vi "Test_Determination_of_Min_Max_Average_Value.vi"() -> ()   [LabVIEW 2022 SP3]
uses:
  SI_modules/SI600/SI600.lvclass
panel:
  out "RCP Spped Loop":cluster{"Time":timestamp[], dbl[]}[](graph)
  out "Inputs":cluster{"Time":timestamp[], dbl[]}[](graph)
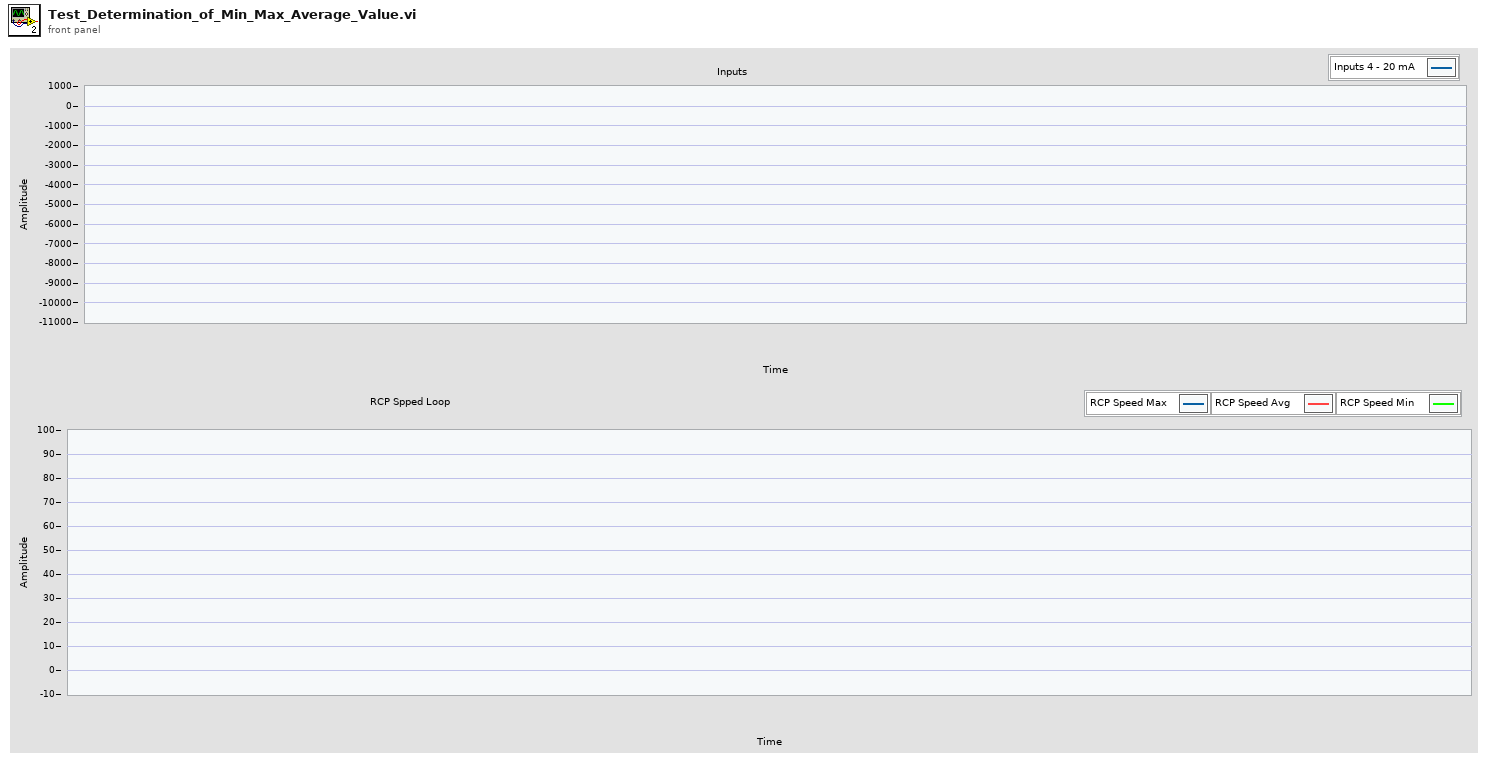
[diagram p1: front panel]
types:
  T1 = cluster{"[0]":cluster{"Time":timestamp[], "KKS":string, "Meas":dbl[]}, "[1]":cluster{"Time":timestamp[], "KKS":string, "Meas":dbl[]}, "[2]":cluster{"Time":timestamp[], "KKS":string, "Meas":dbl[]}, "[3]":cluster{"Time":timestamp[], "KKS":string, "Meas":dbl[]}, "[4]":cluster{"Time":timestamp[], "KKS":string, "Meas":dbl[]}, "[5]":cluster{"Time":timestamp[], "KKS":string, "Meas":dbl[]}, "[6]":cluster{"Time":timestamp[], "KKS":string, "Meas":dbl[]}, "[7]":cluster{"Time":timestamp[], "KKS":string, "Meas":dbl[]}, "[8]":cluster{"Time":timestamp[], "KKS":string, "Meas":dbl[]}}
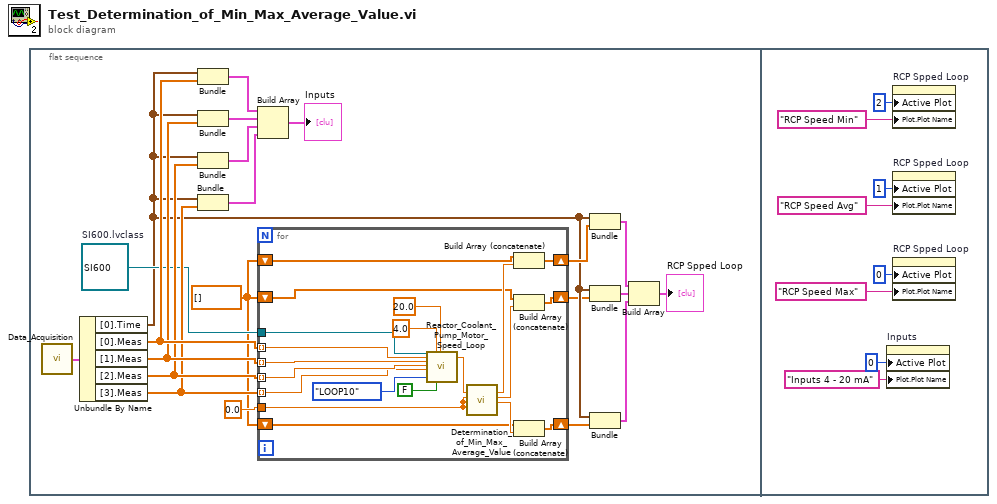
[diagram p0: block diagram]
diagram:
  n1 = flat-sequence {
    frame #0 {
      w11 = refnum<class "SI600.lvclass"> refnum  # SI600.lvclass
      w9 = dbl[] []
      n2 = call "Data_Acquisition.vi"() -> ("Meas"=w21:T1)  [unwired: 15 in]
      n3 = Unbundle By Name(w21) -> ("[0].Time"=w7:timestamp[], "[0].Meas"=w20:dbl[], "[1].Meas"=w19:dbl[], "[2].Meas"=w18:dbl[], "[3].Meas"=w17:dbl[])
      n4 = Bundle("Time"=w7, "Meas"=w20) -> (w16:cluster{"Time":timestamp[], "Meas":dbl[]})  [unwired: 1 in]
      n5 = Bundle("Time"=w7, "Meas"=w19) -> (w15:cluster{"Time":timestamp[], "Meas":dbl[]})  [unwired: 1 in]
      n6 = Bundle("Time"=w7, "Meas"=w18) -> (w14:cluster{"Time":timestamp[], "Meas":dbl[]})  [unwired: 1 in]
      n7 = Bundle("Time"=w7, "Meas"=w17) -> (w13:cluster{"Time":timestamp[], "Meas":dbl[]})  [unwired: 1 in]
      n8 = Build Array(w16, w15, w14, w13) -> (→"Inputs":cluster{"Time":timestamp[], "Meas":dbl[]}[])
      n9 = for {
        tunnel: w11 -> [w41]
        tunnel: w20 -> [w40] mode=indexing
        tunnel: w19 -> [w39] mode=indexing
        tunnel: w18 -> [w38] mode=indexing
        tunnel: w17 -> [w37] mode=indexing
        tunnel: 0.0 ("RCP speed Loop 20") -> [w31]
        shift-right: [w27] -> w8
        shift-left: w9 -> [w24]
        shift-right: [w26] -> w6
        shift-left: w9 -> [w23]
        shift-right: [w25] -> w5
        shift-left: w9 -> [w22]
        n10 = call "Reactor_Coolant_Pump_Motor_Speed_Loop.vi"("SI600.lvclass in"=w41, "3 JEB CS951 XQ01"=w40, "3 JEB CS952 XQ01"=w39, "3 JEB CS953 XQ01"=w38, "3 JEB CS954 XQ01"=w37, "Loop"=enum16{"LOOP10", "LOOP20", "LOOP30", "LOOP40"}."LOOP10", "In1"=4.0, "Limitation"=FALSE, "In2"=20.0) -> ("RCP speed Loop Output"=w32:dbl)  [unwired: 12 in, 6 out]
        n11 = call "Determination_of_Min_Max_Average_Value.vi"("RCP speed Loop 10"=w32, "RCP speed Loop 20"=w31, "RCP speed Loop 30"=w31, "RCP speed Loop 40"=w31) -> ("RCP Speed Max"=w30:dbl, "RCP Speed AVG"=w29:dbl, "RCP Speed Min"=w28:dbl)  [unwired: 11 in, 2 out]
        n12 = Build Array (concatenate)(w24, w30) -> (w27:dbl[])
        n13 = Build Array (concatenate)(w23, w29) -> (w26:dbl[])
        n14 = Build Array (concatenate)(w22, w28) -> (w25:dbl[])
      }
      n15 = Bundle("Time"=w7, w8) -> (w4:cluster{"Time":timestamp[], dbl[]})  [unwired: 1 in]
      n16 = Bundle("Time"=w7, w6) -> (w3:cluster{"Time":timestamp[], dbl[]})  [unwired: 1 in]
      n17 = Bundle("Time"=w7, w5) -> (w2:cluster{"Time":timestamp[], dbl[]})  [unwired: 1 in]
      n18 = Build Array(w4, w3, w2) -> (→"RCP Spped Loop":cluster{"Time":timestamp[], dbl[]}[])
    }
    frame #1 {
      n19 = property on="Inputs" class="XYGraph (strict)"("Active Plot"=u32 0, "Plot.Plot Name"="Inputs 4 - 20 mA") -> ()  [unwired: 2 in, 2 out]
      n20 = property on="RCP Spped Loop" class="XYGraph (strict)"("Active Plot"=u32 2, "Plot.Plot Name"="RCP Speed Min") -> ()  [unwired: 2 in, 2 out]
      n21 = property on="RCP Spped Loop" class="XYGraph (strict)"("Active Plot"=u32 1, "Plot.Plot Name"="RCP Speed Avg") -> ()  [unwired: 2 in, 2 out]
      n22 = property on="RCP Spped Loop" class="XYGraph (strict)"("Active Plot"=u32 0, "Plot.Plot Name"="RCP Speed Max") -> ()  [unwired: 2 in, 2 out]
    }
  }
